vi "RIMAS Detectors Process Image.vi"(5 "Charts":refnum<vi>[](array[refnum]), 7 "Image Refs":refnum<vi>[](array[refnum]), 8 "Force UNSIGNED":bool, 9 "Frame Num":i32, 10 "Detector Num":i32, 11 "FITS file":path) -> (1 "Res file names":path[](array[path]), 2 "Det 2 Files":path[](array[path]), 3 "Det 1 Files":path[](array[path]))   [LabVIEW 2020]
panel:
  in  "Tab Control":enum32{"Page 1", "Page 2"}(tab)
  out "Res file names 2":path[](array[path])
  out "Image  1 - pedestal":sgl[][](graph)
  out "Image  2 signal current":sgl[][](graph)
  out "current signal file name":string
  out "Ref file dir name":path
  out "current signal file name 2":string
  out "Peak 2":sgl[][](graph)
  out "Peak pedesrtal":sgl[][](graph)
  out "Signal dri name":path
  out "Image YJ":dbl[][](graph)
  out "Stdev 2":dbl(graph)
  out "Stdev":dbl(graph)
  out "Image HK":dbl[][](graph)
  out "Fnames YJ":path[](array[path])
  out "Fnames HK":path[](array[path])
  out "Frame 0 HK":dbl[][](array[numeric])
  out "Frame 0 YJ":dbl[][](array[numeric])
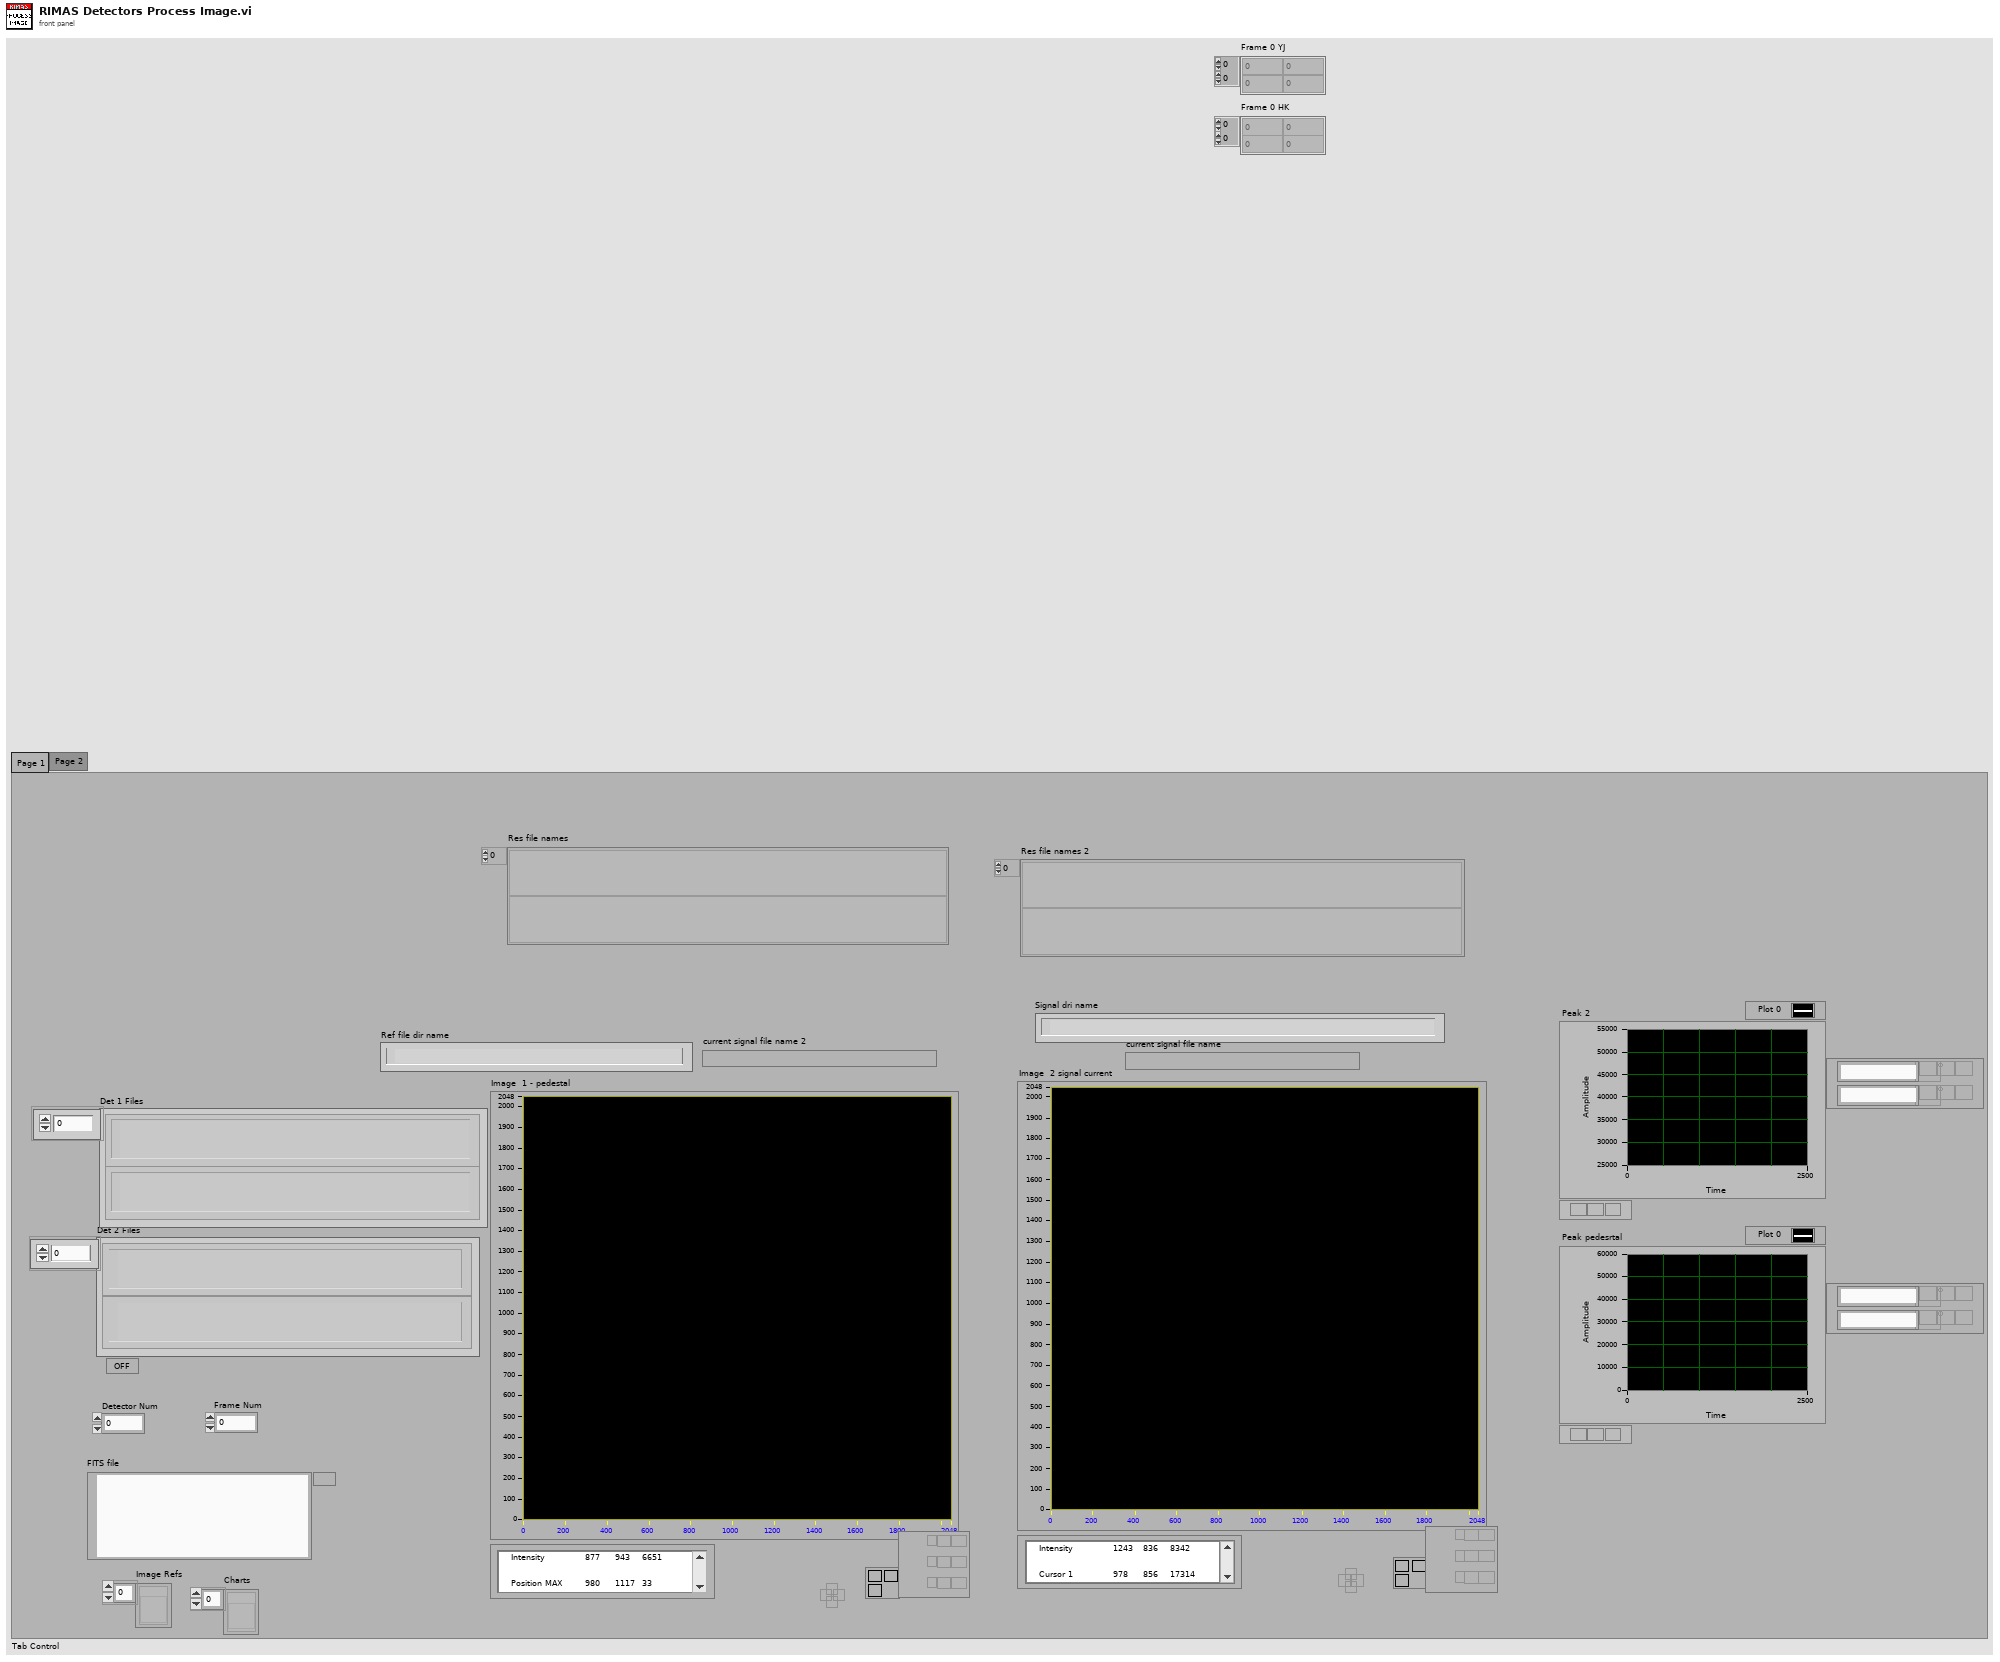
[diagram p1: front panel]
types:
  T1 = cluster{"amplitude":dbl, " center":dbl, " standard deviation":dbl, "offset":dbl}
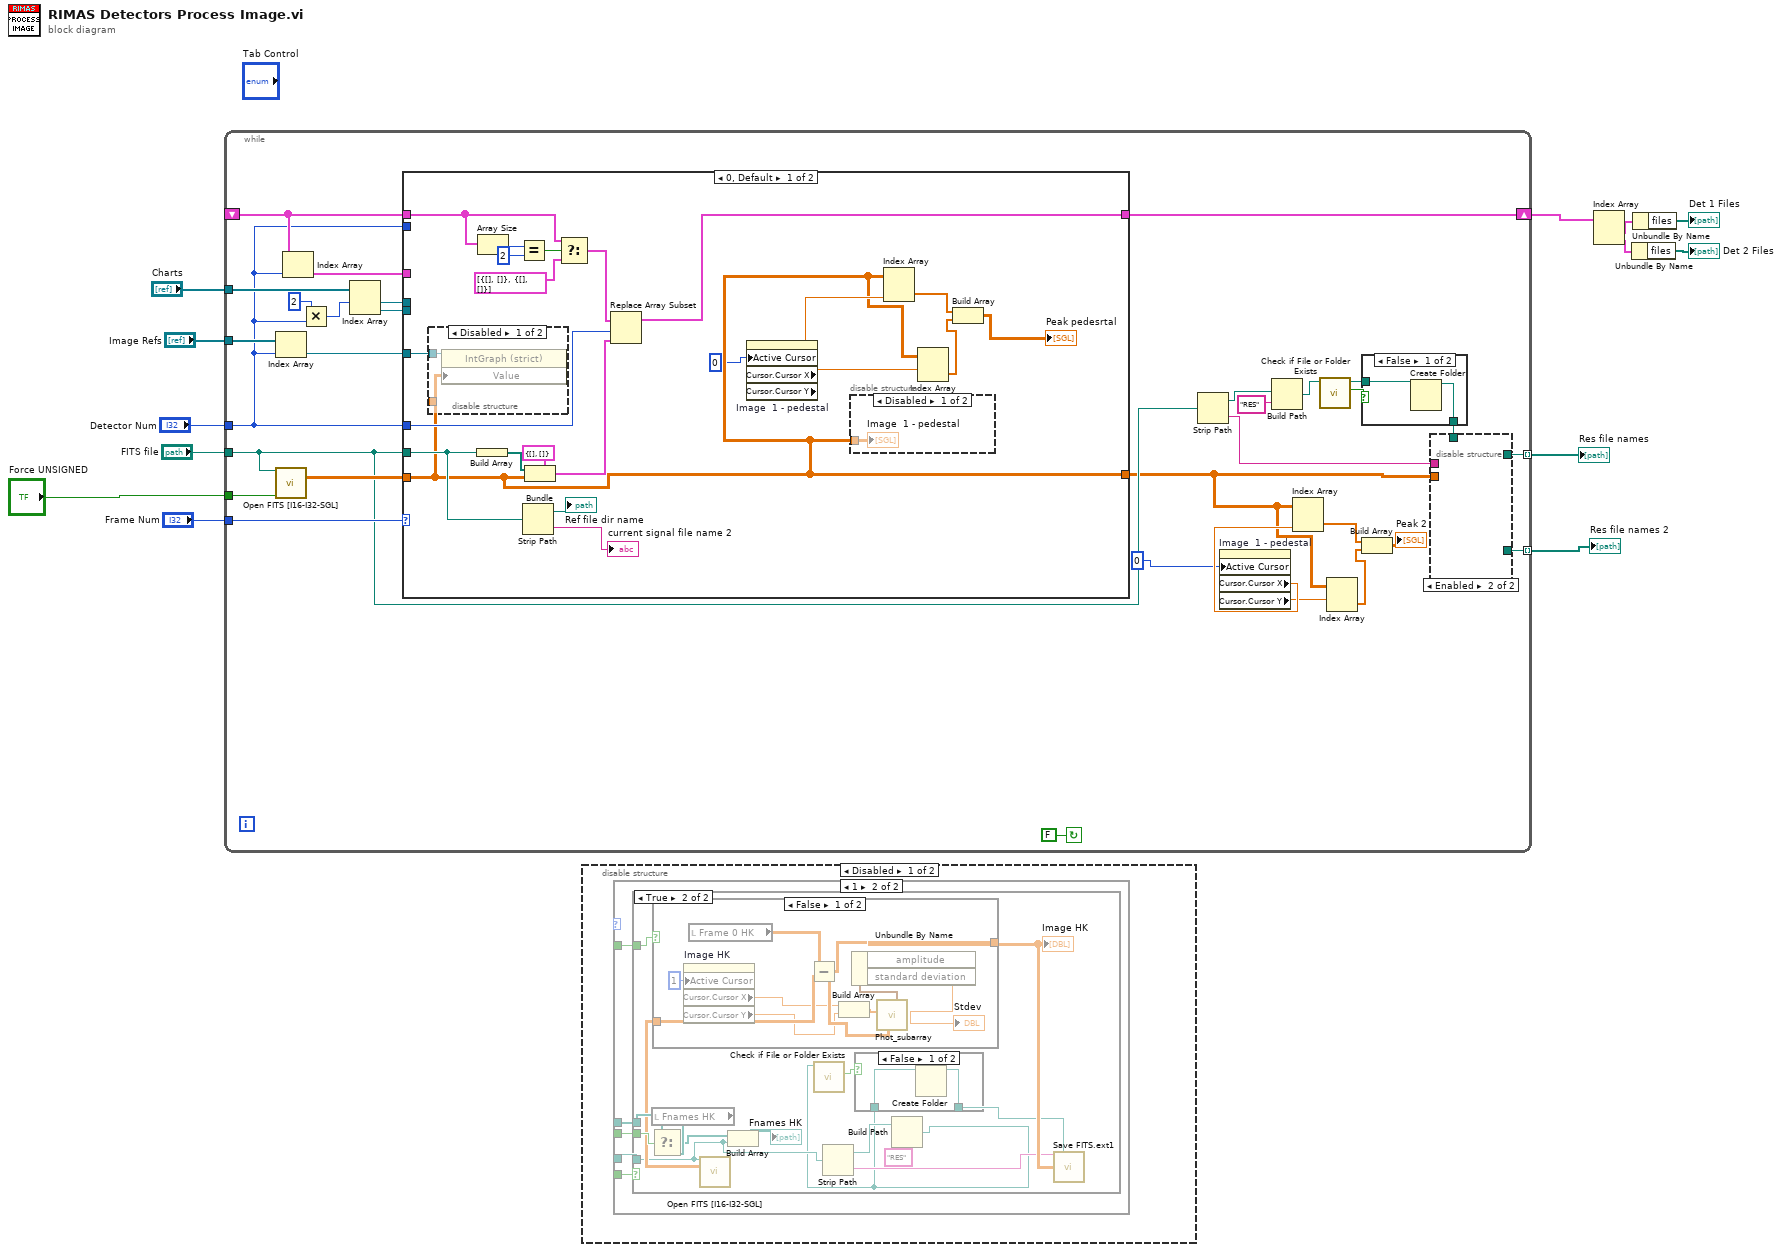
[diagram p0: block diagram]
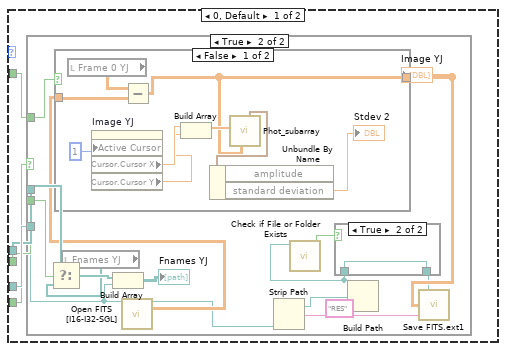
[diagram p2: hidden frame]
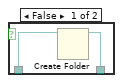
[diagram p4: hidden frame]
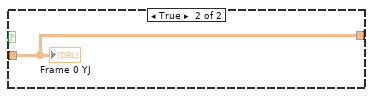
[diagram p5: hidden frame]
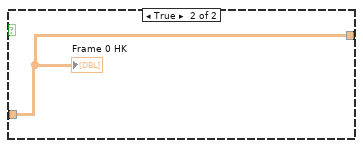
[diagram p8: hidden frame]
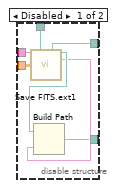
[diagram p10: hidden frame]
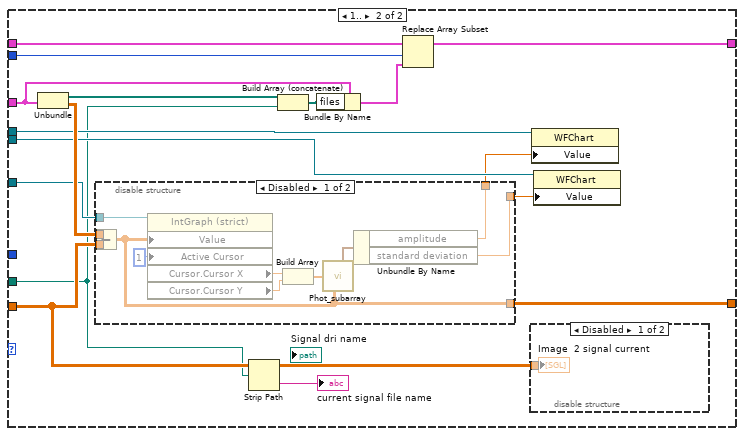
[diagram p14: hidden frame]
diagram:
  n1 = while {
    shift-right: [w43] -> w8
    shift-left: _ -> [w41]
    tunnel: "Frame Num" -> [w45]
    tunnel: "FITS file" -> [w27]
    tunnel: "Detector Num" -> [w32]
    tunnel: "Image Refs" -> [w38]
    tunnel: "Charts" -> [w35]
    tunnel: [w23] -> w3 mode=indexing
    tunnel: [w22] -> w2 mode=indexing
    tunnel: "Force UNSIGNED" -> [w21]
    stop <- FALSE continue-if-true
    n2 = Index Array(array=w38, index=w32) -> (element=w42:refnum<vi>)
    n3 = call "Open FITS [I16-I32-SGL].vi"("Input File:"=w27, 11:w21) -> ("Image"=w44:sgl[][])  [unwired: 11 in, 2 out]
    n4 = Index Array(array=w41, index=w32) -> (element=w40:cluster{"files":path[], "Image0":sgl[][]})
    n5 = Multiply(x=2, y=w32) -> (x*y=w36:i32)
    n6 = Index Array(array=w35, index #1=w36) -> (element #1=w34:refnum<vi>, element #2=w33:refnum<vi>)  [unwired: 1 in]
    n7 = case shown="0, Default" w45 {
      tunnel: w44 -> [w57 w84]
      tunnel: w27 -> [w65 w83]
      tunnel: w32 -> [w75 _]
      tunnel: [w73 w90] -> w43
      tunnel: w41 -> [w69 w93]
      tunnel: w42 -> [w66 w96]
      tunnel: w40 -> [_ w95]
      tunnel: w32 -> [_ w91]
      tunnel: w34 -> [_ w89]
      tunnel: w33 -> [_ w88]
      tunnel: [w57 w85] -> w19
      frame 0, Default {
        n8 = disable-structure shown="Disabled" {
          disable-tunnel: w66 -> [w79 _]
          disable-tunnel: w57 -> [w78 _]
          frame Disabled {
            n9 = property class="IntGraph (strict)"(reference=w79, "Value"=w78) -> ()  [unwired: 1 in, 2 out]
          }
          frame Enabled {
          }
        }
        n10 = Build Array(w65) -> (w77:path[])
        n11 = Array Size(array=w69) -> (size(s)=w72:i32)
        n12 = Equal?(x=w72, y=2) -> (x = y?=w70:bool)
        n13 = Strip Path(path=w65) -> (stripped path=→"Ref file dir name":path, name=→"current signal file name 2":string)
        n14 = Bundle(cluster=cluster{"files":path[], "Image0":sgl[][]} {"files"=[], "Image0"=[]}, "files"=w77, "Image0"=w57) -> (w74:cluster{"files":path[], "Image0":sgl[][]})
        n15 = Select(t=w69, s=w70, f=cluster{"files":path[], "Image0":sgl[][]}[] [{"files"=[], "Image0"=[]}, {"files"=[], "Image0"=[]}]) -> (s? t:f=w67:cluster{"files":path[], "Image0":sgl[][]}[])
        n16 = Replace Array Subset(array=w67, new element=w74, index=w75) -> (w73:cluster{"files":path[], "Image0":sgl[][]}[])
        n17 = property on="Image  1 - pedestal" class="IntGraph (strict)"("Active Cursor"=u32 0) -> ("Cursor.Cursor X"=w61:dbl, "Cursor.Cursor Y"=w60:dbl)  [unwired: 2 in, 2 out]
        n18 = disable-structure shown="Disabled" {
          disable-tunnel: w57 -> [w80 _]
          frame Disabled {
            "Image  1 - pedestal" <- w80
          }
          frame Enabled {
          }
        }
        n19 = Index Array(array=w57, index (col)=w61) -> (element=w59:sgl[])  [unwired: 1 in]
        n20 = Index Array(array=w57, index (row)=w60) -> (element=w58:sgl[])  [unwired: 1 in]
        n21 = Build Array(w59, w58) -> (→"Peak pedesrtal":sgl[][])
      }
      frame 1.. {
        n22 = Unbundle(w95) -> ("files"=w98:path[], "Image0"=w97:sgl[][])
        n23 = disable-structure shown="Disabled" {
          disable-tunnel: w97 -> [w110 _]
          disable-tunnel: w96 -> [w109 _]
          disable-tunnel: [w103 _] -> w87
          disable-tunnel: [w102 _] -> w86
          disable-tunnel: [w101 _] -> w85
          disable-tunnel: w84 -> [w100 _]
          frame Disabled {
            n24 = Subtract(x=w110, y=w100) -> (x-y=w101:sgl[][])
            n25 = property class="IntGraph (strict)"(reference=w109, "Value"=w101, "Active Cursor"=u32 1) -> ("Cursor.Cursor X"=w107:dbl, "Cursor.Cursor Y"=w106:dbl)  [unwired: 1 in, 2 out]
            n26 = Build Array(w107, w106) -> (w105:dbl[])
            n27 = call "Phot_subarray.vi"("Image in"=w101, "XY center"=w105) -> ("Fit Result"=w104:T1)  [unwired: 8 in, 1 out]
            n28 = Unbundle By Name(w104) -> ("amplitude"=w103:dbl, "standard deviation"=w102:dbl)
          }
          frame Enabled {
          }
        }
        n29 = Strip Path(path=w83) -> (stripped path=→"Signal dri name":path, name=→"current signal file name":string)
        n30 = Build Array (concatenate)(w98, w83) -> (w94:path[])
        n31 = Bundle By Name(cluster=w95, "files"=w94) -> (w92:cluster{"files":path[], "Image0":sgl[][]})
        n32 = Replace Array Subset(array=w93, new element=w92, index=w91) -> (w90:cluster{"files":path[], "Image0":sgl[][]}[])
        n33 = disable-structure shown="Disabled" {
          disable-tunnel: w84 -> [w99 _]
          frame Disabled {
            "Image  2 signal current" <- w99
          }
          frame Enabled {
          }
        }
        n34 = property class="WFChart"(reference=w89, "Value"=w87) -> ()  [unwired: 1 in, 2 out]
        n35 = property class="WFChart"(reference=w88, "Value"=w86) -> ()  [unwired: 1 in, 2 out]
      }
    }
    n36 = Strip Path(path=w27) -> (stripped path=w31:path, name=w29:string)
    n37 = property on="Image  1 - pedestal" class="IntGraph (strict)"("Active Cursor"=u32 0) -> ("Cursor.Cursor X"=w20:dbl, "Cursor.Cursor Y"=w18:dbl)  [unwired: 2 in, 2 out]
    n38 = Build Path(base path=w31, name or relative path="RES") -> (appended path=w26:path)
    n39 = Index Array(array=w19, index (col)=w20) -> (element=w17:sgl[])  [unwired: 1 in]
    n40 = call <vilib>:"Check if File or Folder Exists.vi"("path"=w26) -> ("file or folder exists?"=w28:bool, "dup path"=w25:path)  [unwired: 8 in, 1 out]
    n41 = Index Array(array=w19, index (row)=w18) -> (element=w16:sgl[])  [unwired: 1 in]
    n42 = case shown="False" w28 {
      tunnel: [w54 w55] -> w24
      tunnel: w25 -> [w53 w55]
      frame False {
        n43 = Create Folder(path (use dialog)=w53) -> (created path=w54:path)  [unwired: 2 in, 2 out]
      }
      frame True {
      }
    }
    n44 = Build Array(w17, w16) -> (→"Peak 2":sgl[][])
    n45 = disable-structure shown="Enabled" {
      disable-tunnel: w29 -> [w52 _]
      disable-tunnel: w24 -> [w51 _]
      disable-tunnel: [w50 _] -> w23
      disable-tunnel: [w47 _] -> w22
      disable-tunnel: w19 -> [w46 _]
      frame Disabled {
        n46 = call "Save FITS.ext1.vi"("Input Filename:"=w52, "Default Save Directory"=w51, "Array"=w46) -> ("Full file name"=w50:path, "directory Written:"=w49:path, "File written"=w48:string)  [unwired: 8 in, 2 out]
        n47 = Build Path(base path=w49, name or relative path=w48) -> (appended path=w47:path)
      }
      frame Enabled {
      }
    }
  }
  "Res file names" <- w3
  "Res file names 2" <- w2
  n48 = disable-structure shown="Disabled" {
    frame Disabled {
      n49 = case shown="1" {
        selector: _ -> [_ _]
        tunnel: _ -> [w111 w145]
        tunnel: _ -> [w115 w149]
        tunnel: _ -> [w113 w148]
        tunnel: _ -> [w114 w146]
        tunnel: _ -> [w112 w147]
        frame 0, Default {
          n50 = case shown="True" w113 {
            tunnel: w115 -> [_ w120]
            tunnel: w114 -> [_ w127]
            tunnel: w112 -> [_ w128]
            tunnel: w111 -> [_ w124]
            frame False {
            }
            frame True {
              n51 = local read "Fnames YJ"() -> (w126:path[])
              n52 = Select(t=w127, s=w128, f=w126) -> (s? t:f=w129:path[])
              n53 = Build Array(w129, w120) -> (→"Fnames YJ":path[][])
              n54 = call "Open FITS [I16-I32-SGL].vi"("Input File:"=w120) -> ("Image"=w125:sgl[][])  [unwired: 12 in, 2 out]
              n55 = case shown="False" w124 {
                tunnel: w125 -> [w142 w144]
                tunnel: [w134 w144] -> w119
                frame False {
                  n56 = local read "Frame 0 YJ"() -> (w143:dbl[][])
                  n57 = property on="Image YJ" class="IntGraph (strict)"("Active Cursor"=u32 1) -> ("Cursor.Cursor X"=w137:dbl, "Cursor.Cursor Y"=w136:dbl)  [unwired: 2 in, 2 out]
                  n58 = Subtract(x=w143, y=w142) -> (x-y=w134:dbl[][])
                  n59 = Build Array(w137, w136) -> (w138:dbl[])
                  n60 = call "Phot_subarray.vi"("Image in"=w134, "XY center"=w138) -> ("Fit Result"=w135:T1)  [unwired: 8 in, 1 out]
                  n61 = Unbundle By Name(w135) -> ("amplitude"=w140:dbl, "standard deviation"=→"Stdev 2":dbl)
                }
                frame True {
                  "Frame 0 YJ" <- w144
                }
              }
              "Image YJ" <- w119
              n62 = Strip Path(path=w120) -> (stripped path=w123:path, name=w121:string)
              n63 = Build Path(base path=w123, name or relative path="RES") -> (appended path=w117:path)
              n64 = call <vilib>:"Check if File or Folder Exists.vi"("path"=w117) -> ("file or folder exists?"=w118:bool)  [unwired: 8 in, 2 out]
              n65 = case shown="True" w118 {
                tunnel: w117 -> [w132 w133]
                tunnel: [w131 w133] -> w116
                frame False {
                  n66 = Create Folder(path (use dialog)=w132) -> (created path=w131:path)  [unwired: 2 in, 2 out]
                }
                frame True {
                }
              }
              n67 = call "Save FITS.ext1.vi"("Input Filename:"=w121, "Default Save Directory"=w116, "Array"=w119) -> ()  [unwired: 8 in, 5 out]
            }
          }
        }
        frame 1 {
          n68 = case shown="True" w148 {
            tunnel: w149 -> [_ w156]
            tunnel: w147 -> [_ w163]
            tunnel: w146 -> [_ w161]
            tunnel: w145 -> [_ w158]
            frame False {
            }
            frame True {
              n69 = local read "Fnames HK"() -> (w162:path[])
              n70 = Select(t=w161, s=w163, f=w162) -> (s? t:f=w160:path[])
              n71 = call "Open FITS [I16-I32-SGL].vi"("Input File:"=w156) -> ("Image"=w159:sgl[][])  [unwired: 12 in, 2 out]
              n72 = case shown="False" w158 {
                tunnel: w159 -> [w175 w177]
                tunnel: [w172 w177] -> w157
                frame False {
                  n73 = property on="Image HK" class="IntGraph (strict)"("Active Cursor"=u32 1) -> ("Cursor.Cursor X"=w170:dbl, "Cursor.Cursor Y"=w169:dbl)  [unwired: 2 in, 2 out]
                  n74 = local read "Frame 0 HK"() -> (w176:dbl[][])
                  n75 = Subtract(x=w176, y=w175) -> (x-y=w172:dbl[][])
                  n76 = Build Array(w170, w169) -> (w168:dbl[])
                  n77 = call "Phot_subarray.vi"("Image in"=w172, "XY center"=w168) -> ("Fit Result"=w173:T1)  [unwired: 8 in, 1 out]
                  n78 = Unbundle By Name(w173) -> ("standard deviation"=→"Stdev":dbl)  [unwired: 1 out]
                }
                frame True {
                  "Frame 0 HK" <- w177
                }
              }
              "Image HK" <- w157
              n79 = Build Array(w160, w156) -> (→"Fnames HK":path[][])
              n80 = Strip Path(path=w156) -> (stripped path=w155:path, name=w153:string)
              n81 = Build Path(base path=w155, name or relative path="RES") -> (appended path=w150:path)
              n82 = call <vilib>:"Check if File or Folder Exists.vi"("path"=w150) -> ("file or folder exists?"=w152:bool)  [unwired: 8 in, 2 out]
              n83 = case shown="False" w152 {
                tunnel: w150 -> [w166 w167]
                tunnel: [w165 w167] -> w151
                frame False {
                  n84 = Create Folder(path (use dialog)=w166) -> (created path=w165:path)  [unwired: 2 in, 2 out]
                }
                frame True {
                }
              }
              n85 = call "Save FITS.ext1.vi"("Input Filename:"=w153, "Default Save Directory"=w151, "Array"=w157) -> ()  [unwired: 8 in, 5 out]
            }
          }
        }
      }
    }
    frame Enabled {
    }
  }
  n86 = Index Array(array=w8) -> (element #1=w7:cluster{"files":path[], "Image0":sgl[][]}, element #2=w6:cluster{"files":path[], "Image0":sgl[][]})  [unwired: 2 in]
  n87 = Unbundle By Name(w6) -> ("files"=→"Det 2 Files":path[])
  n88 = Unbundle By Name(w7) -> ("files"=→"Det 1 Files":path[])
